vi "CloseXL_App.vi"(8 "error in (no error)":errorcluster, 11 "Refnum Cluster In":T1) -> (0 "error out":errorcluster)   [LabVIEW 2017, in "excel_configuration.lvlib"]
doc: "Closes the Excel application reference opened by OpenXL_App.vi."
uses:
  excel_configuration.lvlib
  1a087639-cb7d-476e-a346-349dcbf1591b.vi
  40add39f-2062-4ef0-94a6-24f3aa9dbb8b.vi
  <vilib>/Utility/error.llb/Clear Errors.vi
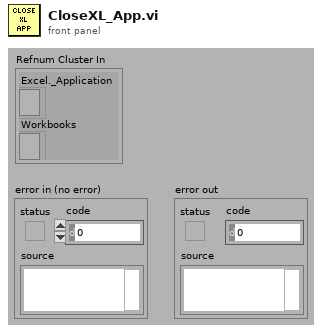
[diagram p1: front panel]
types:
  T1 = cluster{"Excel._Application":refnum<k7>, "Workbooks":refnum<k7>}
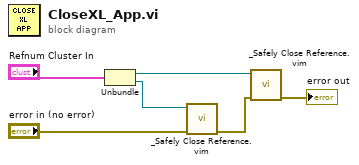
[diagram p0: block diagram]
diagram:
  n1 = Unbundle("Refnum Cluster In") -> ("Excel._Application"=w3:refnum<k7>, "Workbooks"=w2:refnum<k7>)
  n2 = call "_Safely Close Reference.vim"("error in (no error)"="error in (no error)", "Automation Refnum in"=w2) -> ("error out"=w4:errorcluster)  [unwired: 9 in]
  n3 = call "_Safely Close Reference.vim"("error in (no error)"=w4, "Automation Refnum in"=w3) -> ("error out"=→"error out":errorcluster)  [unwired: 9 in]
